vi "MPS_Feedback_Spec.vi"(0 "Ref mT":dbl=10.214925362492602, 3 "Expected mT Spec Drive":dbl=10.978070113026728 format="%#_7p", 5 "last N array":dbl[](array[numeric])=[10.978070113026728, 10.214925362492602] format="%#_6p", 9 "Error Gain":dbl=1.0, 11 "Loop num":i32=5, 12 "Num avgs":i32=2) -> (1 "Relative Drive":dbl=-26.770610307790598, 4 "Updated Tx Amp":dbl=nan, 14 "Error":dbl=-0.3815723752670639, 15 "Updated last N":dbl[](array[numeric])=[10.978070113026728, 10.214925362492602])   [LabVIEW 2021]
uses:
  <vilib>/Analysis/1siggen.llb/Ramp Pattern by Samples.vi
  <vilib>/Analysis/baseanly.llb/Mean (DBL).vi
  MPS_global_variables.vi
  <vilib>/Analysis/NI_AALBase.lvlib
panel:
  out "x/y":dbl
  out "Ramp Pattern":dbl[](array[numeric])
  in  "Triangular\nWeighting?":bool=TRUE
  out "x-y*floor(x/y)":i32
  out "Correction factor":dbl
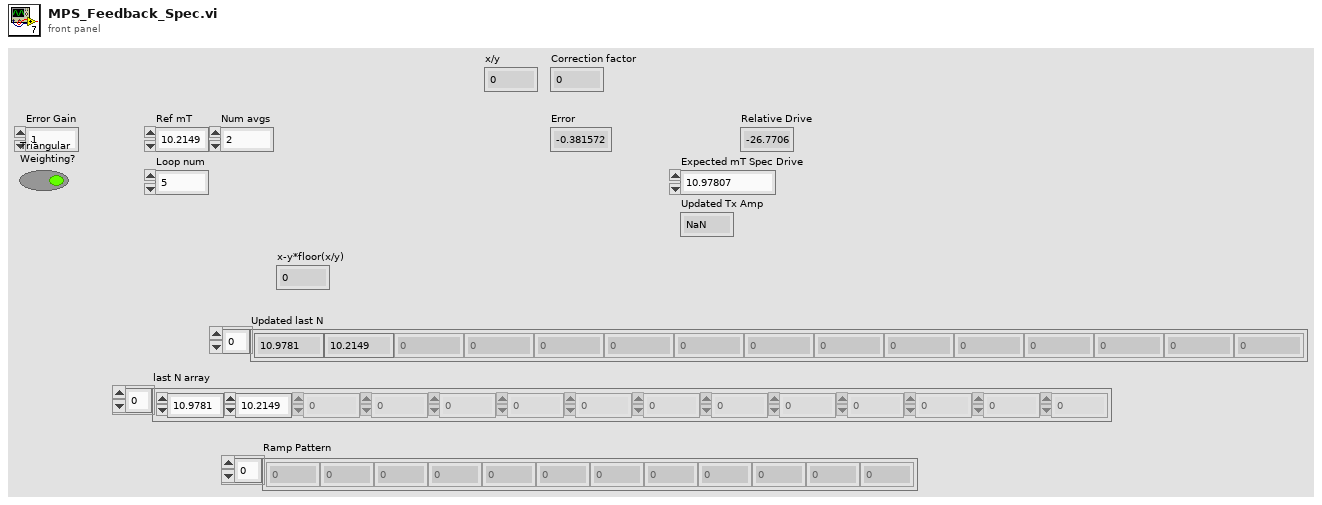
[diagram p1: front panel]
types:
  T1 = cluster{"sample rate":dbl, "Tx freq":dbl, "Tx amp":dbl, "Tx cycles\nSpectroscopy":dbl, "Bias amp":dbl, "Bias freq":dbl, "Receive range":dbl, "Bias Periods\nMagnetometry":dbl, "Tx Freq Division Factor":dbl, "Drive Periods per Bias":dbl, "TX harmonics":dbl[]}
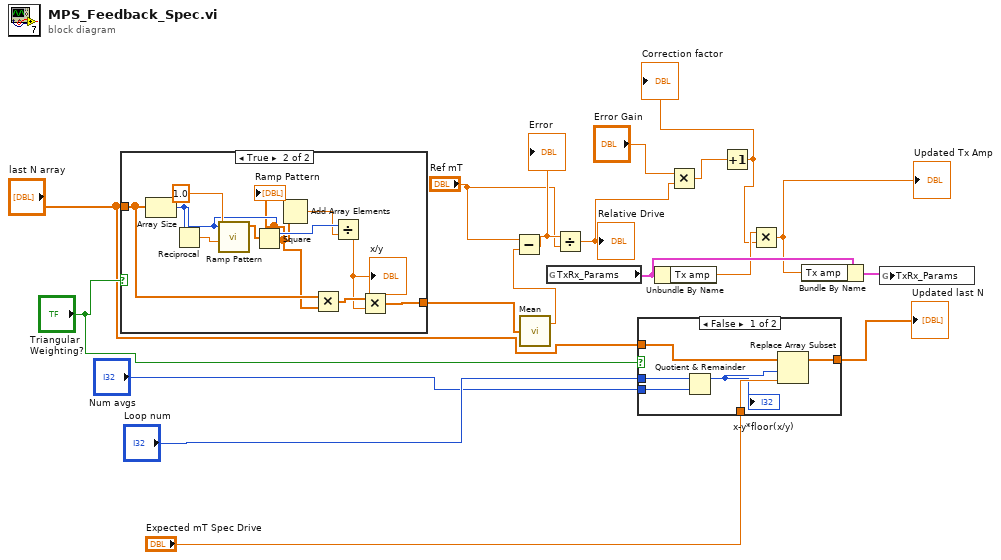
[diagram p0: block diagram]
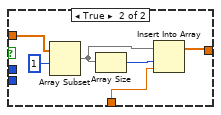
[diagram p3: hidden frame]
diagram:
  n1 = case shown="True" "Triangular\nWeighting?" {
    tunnel: "last N array" -> [w19 w27]
    tunnel: [w19 w25] -> w3
    frame False {
    }
    frame True {
      n2 = Array Size(array=w27) -> (size(s)=w24:i32)
      n3 = Reciprocal(x=w24) -> (1/x=w28:dbl)
      n4 = call-poly <vilib>:"Ramp Pattern.vi"("start"=w28, "end"=1.0, "samples"=w24) -> ("Ramp Pattern"=w21:dbl[])  [unwired: 7 in, 1 out]
      n5 = Square(x=w21) -> (x^2=w20:dbl[])
      "Ramp Pattern" <- w20
      n6 = Add Array Elements(numeric array=w20) -> (sum=w23:dbl)
      n7 = Multiply(x=w27, y=w20) -> (x*y=w26:dbl[])
      n8 = Divide(x=w24, y=w23) -> (x/y=w22:dbl)
      "x/y" <- w22
      n9 = Multiply(x=w26, y=w22) -> (x*y=w25:dbl[])
    }
  }
  n10 = call-poly <vilib>:"Mean.vi"("X"=w3) -> ("mean"=w11:dbl)  [unwired: 1 out]
  n11 = Subtract(x="Ref mT", y=w11) -> (x-y=w10:dbl)
  "Error" <- w10
  n12 = global read "MPS_global_variables.vi" "TxRx_Params"() -> (w18:T1)
  n13 = Divide(x=w10, y="Ref mT") -> (x/y=w4:dbl)
  "Relative Drive" <- w4
  n14 = case shown="False" "Triangular\nWeighting?" {
    tunnel: "Expected mT Spec Drive" -> [w35 w39]
    tunnel: [w34 w38] -> w13
    tunnel: "Loop num" -> [w32 _]
    tunnel: "Num avgs" -> [w31 _]
    tunnel: "last N array" -> [w30 w37]
    frame False {
      n15 = Quotient & Remainder(x=w32, y=w31) -> (x-y*floor(x/y)=w33:i32)  [unwired: 1 out]
      "x-y*floor(x/y)" <- w33
      n16 = Replace Array Subset(array=w30, new element=w35, index=w33) -> (w34:dbl[])
    }
    frame True {
      n17 = Array Subset(array=w37, index=1) -> (w36:dbl[])  [unwired: 1 in]
      n18 = Array Size(array=w36) -> (size(s)=w40:i32)
      n19 = Insert Into Array(array=w36, index=w40, new element=w39) -> (w38:dbl[])
    }
  }
  "Updated last N" <- w13
  n20 = Unbundle By Name(w18) -> ("Tx amp"=w15:dbl)
  n21 = Multiply(x="Error Gain", y=w4) -> (x*y=w6:dbl)
  n22 = Increment(x=w6) -> (x+1=w5:dbl)
  "Correction factor" <- w5
  n23 = Multiply(x=w15, y=w5) -> (x*y=w16:dbl)
  "Updated Tx Amp" <- w16
  n24 = Bundle By Name(cluster=w18, "Tx amp"=w16) -> (w17:T1)
  n25 = global write "MPS_global_variables.vi" "TxRx_Params"(w17) -> ()
